vi "LigthUpGameboard.vi"(8 "error in (no error)":errorcluster, 10 "Indices":i8[](array[numeric]), 11 "Button Refs":refnum<vi>[](array[refnum])) -> (0 "error out":errorcluster)   [LabVIEW 2020]
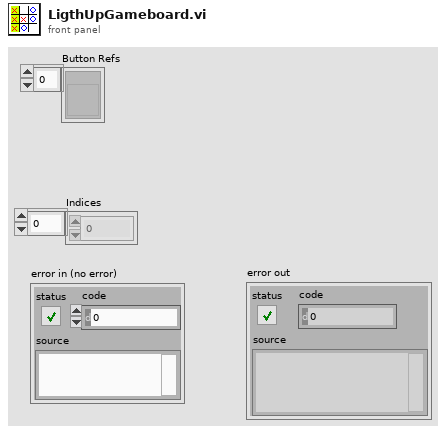
[diagram p1: front panel]
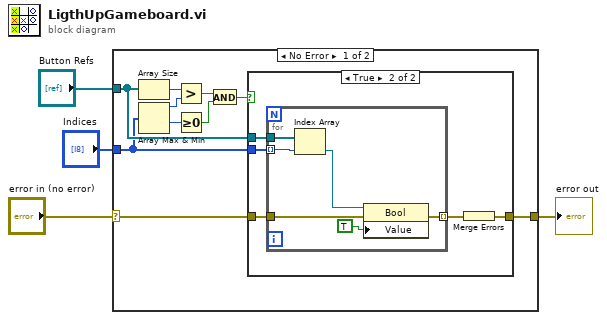
[diagram p0: block diagram]
diagram:
  n1 = case shown="No Error" "error in (no error)" {
    selector: "error in (no error)" -> [w14 w27]
    tunnel: [w5 w27] -> w3
    tunnel: "Indices" -> [w12 _]
    tunnel: "Button Refs" -> [w13 _]
    frame No Error {
      n2 = Array Size(array=w13) -> (size(s)=w10:i32)
      n3 = Array Max & Min(array=w12) -> (max value=w9:i8, min value=w11:i8)  [unwired: 2 out]
      n4 = Greater?(x=w10, y=w9) -> (0:w7:bool)
      n5 = Greater Or Equal To 0?(x=w11) -> (x >= 0?=w8:bool)
      n6 = And(x=w7, y=w8) -> (x .and. y?=w6:bool)
      n7 = case shown="True" w6 {
        tunnel: w12 -> [_ w20]
        tunnel: w13 -> [_ w19]
        tunnel: w14 -> [w15 w18]
        tunnel: [w15 w16] -> w5
        frame False {
        }
        frame True {
          n8 = for {
            tunnel: w20 -> [w25] mode=indexing
            tunnel: w19 -> [w26]
            tunnel: w18 -> [w23]
            tunnel: [w22] -> w17 mode=indexing
            n9 = Index Array(array=w26, index=w25) -> (element=w24:refnum<vi>)
            n10 = property class="Bool"(reference=w24, error in=w23, "Value"=TRUE) -> (error out=w22:errorcluster)  [unwired: 1 out]
          }
          n11 = Merge Errors(w17) -> (w16:errorcluster)
        }
      }
    }
    frame Error {
    }
  }
  "error out" <- w3
